vi "PathPlanner_PathFinder_WorkerThread.vi"() -> ()   [LabVIEW 2019]
uses:
  PathPlannerLib24/VI/PathPlanner_GridPosition_New.vi
  PathPlannerLib24/VI/PathPlanner_GridPosition_HashCode.vi
  PathPlannerLib24/VI/PathPlanner_PathFinder_Constants.vi
  PathPlannerLib24/VI/PathPlanner_PathFinder_Key.vi
  PathPlannerLib24/VI/PathPlanner_PathFinder_ClearOpen.vi
  PathPlannerLib24/VI/PathPlanner_PathFinder_ClearIncons.vi
  PathPlannerLib24/VI/PathPlanner_PathFinder_ClearClosed.vi
  PathPlannerLib24/VI/PathPlanner_PathFinder_ClearRHS.vi
  PathPlannerLib24/VI/PathPlanner_PathFinder_ClearG.vi
  PathPlannerLib24/VI/PathPlanner_PathFinder_ComputeOrImprovePath.vi
  PathPlannerLib24/VI/PathPlanner_PathFinder_SetNewPathAvail.vi
  PathPlannerLib24/VI/PathPlanner_PathFinder_ExtractPath.vi
  PathPlannerLib24/VI/PathPlanner_GridPosition_FromHash.vi
  PathPlannerLib24/VI/PathPlanner_GridPosition_Get.vi
  PathPlannerLib24/VI/PathPlanner_PathFinder_Heuristic.vi
  PathPlannerLib24/VI/PathPlanner_PathFinder_TopKey.vi
  PathPlannerLib24/VI/PathPlanner_PathFinder_ComparePair.vi
  PathPlannerLib24/VI/PathPlanner_PathFinder_UpdateState.vi
  PathPlannerLib24/VI/PathPlanner_PathFinder_GetOpenNeighbors.vi
  PathPlannerLib24/VI/PathPlanner_GridPosition_Equals.vi
  PathPlannerLib24/VI/PathPlanner_PathFinder_GridPosToTranslation2d.vi
  <vilib>/Rock Robotics/WPI/ThirdParty/JAS_Junk/TrajLib/Translation2d_GetDistance.vi
  <vilib>/Rock Robotics/WPI/ThirdParty/JAS_Junk/TrajLib/Translation2d_Create_DistAng.vi
  <vilib>/Rock Robotics/WPI/ThirdParty/JAS_Junk/TrajLib/Translation2d_Minus.vi
  <vilib>/Rock Robotics/WPI/ThirdParty/JAS_Junk/TrajLib/Translation2d_GetAngle.vi
  <vilib>/Rock Robotics/WPI/ThirdParty/JAS_Junk/TrajLib/Translation2d_Plus.vi
  PathPlannerLib24/VI/PathPlanner_PathFinder_ExtractPathSub1ALT.vi
  PathPlannerLib24/VI/PathPlanner_PathFinder_IsWalkable.vi
  PathPlannerLib24/VI/PathPlanner_PathFinder_Cost.vi
  <vilib>/Rock Robotics/WPI/ThirdParty/JAS_Junk/TrajLib/Translation2d_Create.vi
  <vilib>/Rock Robotics/WPI/ThirdParty/JAS_Junk/TrajLib/Util_CalcDist.vi
  <vilib>/Rock Robotics/WPI/ThirdParty/JAS_Junk/TrajLib/Rotation2d_GetAngleCosSin.vi
  <vilib>/Rock Robotics/WPI/ThirdParty/JAS_Junk/TrajLib/Translation2d_GetXY.vi
  <vilib>/Rock Robotics/WPI/ThirdParty/JAS_Junk/TrajLib/Rotation2d_CreateXY.vi
  PathPlannerLib24/VI/PathPlanner_PathFinder_IsCollision.vi
  PathPlannerLib24/VI/PathPlanner_GridPosition_Print.vi
  <vilib>/robotics/Navigation/shared/MapNode/AbstractDstarNode/NI_Robotics_AbstractDstarNode.lvclass
  C:/Program Files/National Instruments/LabVIEW 2019/vi.lib/robotics/Navigation/shared/MapNode/AbstractAstarNode/NI_Robotics_AbstractAstarNode.lvclass
  PathPlannerLib24/VI/PathPlanner_PathFinder_Globals.vi
  <vilib>/robotics/Navigation/shared/WorldMap/OccupancyGridWorldMap/Get Cells in Path.vi
  PathPlannerLib24/VI/PathPlanner_PathFinder_ApplyControlSmooth.vi
  PathPlannerLib24/VI/PathPlanner_PathFinder_ApplyAnchorSmooth.vi
  PathPlannerLib24/PathPlanner24.lvlib
panel:
  in  "Main Name":string
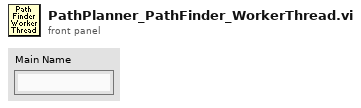
[diagram p1: front panel]
types:
  T1 = typedef "Semaphore RefNum" = refnum<k1>
  T2 = enum32{"Bad", "Idle", "Run top level", "Running"}
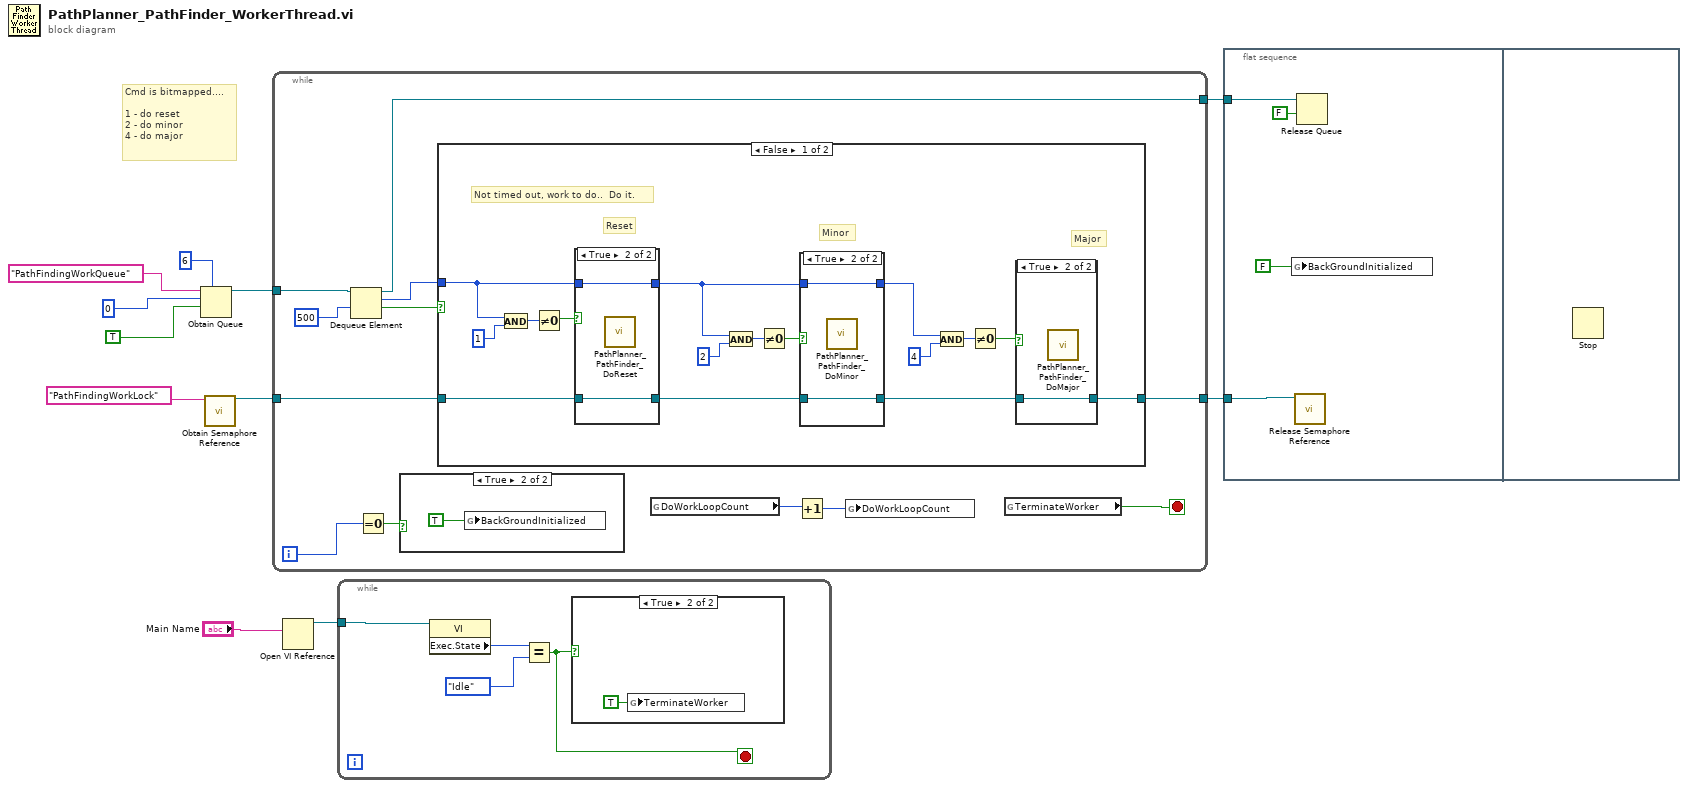
[diagram p0: block diagram]
diagram:
  # "Cmd is bitmapped....\n\n1 - do reset\n2 - do minor\n4 - do major"
  n1 = Obtain Queue(max queue size (-1, unlimited)=6, name (unnamed)="PathFindingWorkQueue", element data type=0, create if not found? (T)=TRUE) -> (queue out=w3:refnum<queue>)  [unwired: 1 in, 2 out]
  n2 = call <vilib>:"Obtain Semaphore Reference.vi"("name (unnamed)"="PathFindingWorkLock") -> ("semaphore"=w5:T1)  [unwired: 4 in, 2 out]
  n3 = while {
    tunnel: w3 -> [w22]
    tunnel: [w18] -> w7
    tunnel: w5 -> [w17]
    tunnel: [w16] -> w4
    i -> [w13]
    stop <- w23 stop-if-true
    n4 = Dequeue Element(queue=w22, timeout in ms (-1)=500) -> (queue out=w18:refnum<queue>, element=w19:i32, timed out?=w20:bool)  [unwired: 1 in, 1 out]
    n5 = Equal To 0?(x=w13) -> (x = 0?=w12:bool)
    n6 = case shown="True" w12 {
      frame False {
      }
      frame True {
        n7 = global write "PathPlanner_PathFinder_Globals.vi" "BackGroundInitialized"(TRUE ("TerminateWorker")) -> ()
      }
    }
    n8 = case shown="False" w20 {
      tunnel: w19 -> [w35 _]
      tunnel: w17 -> [w28 w51]
      tunnel: [w25 w51] -> w16
      frame False {
        # "Major"
        # "Minor"
        # "Reset"
        # "Not timed out, work to do..  Do it."
        n9 = And(x=w35, y=1) -> (x .and. y?=w38:i32)
        n10 = Not Equal To 0?(x=w38) -> (x != 0?=w39:bool)
        n11 = case shown="True" w39 {
          tunnel: w35 -> [w48 w50]
          tunnel: [w48 w50] -> w31
          tunnel: w28 -> [w47 w49]
          tunnel: [w47 w49] -> w27
          frame False {
          }
          frame True {
            n12 = call "PathPlanner_PathFinder_DoReset.vi"() -> ()  [unwired: 12 in]
          }
        }
        n13 = And(x=w31, y=2) -> (x .and. y?=w36:i32)
        n14 = Not Equal To 0?(x=w36) -> (x != 0?=w32:bool)
        n15 = case shown="True" w32 {
          tunnel: w31 -> [w44 w46]
          tunnel: [w44 w46] -> w29
          tunnel: w27 -> [w43 w45]
          tunnel: [w43 w45] -> w26
          frame False {
          }
          frame True {
            n16 = call "PathPlanner_PathFinder_DoMinor.vi"() -> ()  [unwired: 12 in]
          }
        }
        n17 = And(x=w29, y=4) -> (x .and. y?=w33:i32)
        n18 = Not Equal To 0?(x=w33) -> (x != 0?=w30:bool)
        n19 = case shown="True" w30 {
          tunnel: w26 -> [w41 w42]
          tunnel: [w41 w42] -> w25
          frame False {
          }
          frame True {
            n20 = call "PathPlanner_PathFinder_DoMajor.vi"() -> ()  [unwired: 12 in]
          }
        }
      }
      frame True {
        # "#TODO  Add I'm alive counter"
        # "Timed out, no work to do...."
      }
    }
    n21 = global read "PathPlanner_PathFinder_Globals.vi" "DoWorkLoopCount"() -> (w15:i64)
    n22 = Increment(x=w15) -> (x+1=w14:i64)
    n23 = global write "PathPlanner_PathFinder_Globals.vi" "DoWorkLoopCount"(w14) -> ()
    n24 = global read "PathPlanner_PathFinder_Globals.vi" "TerminateWorker"() -> (w23:bool)
  }
  n25 = Open VI Reference(vi path="Main Name") -> (vi reference=w1:refnum<vi>)  [unwired: 5 in, 1 out]
  n26 = while {
    tunnel: w1 -> [w52]
    stop <- w53 stop-if-true
    n27 = property class="VI"(reference=w52) -> ("Exec.State"=w55:T2)  [unwired: 1 in, 2 out]
    n28 = Equal?(x=w55, y=T2."Idle") -> (x = y?=w53:bool)
    n29 = case shown="True" w53 {
      frame False {
      }
      frame True {
        n30 = global write "PathPlanner_PathFinder_Globals.vi" "TerminateWorker"(TRUE ("TerminateWorker")) -> ()
      }
    }
  }
  n31 = flat-sequence {
    tunnel: w7 -> [w60]
    tunnel: w4 -> [w58]
    frame #0 {
      n32 = global write "PathPlanner_PathFinder_Globals.vi" "BackGroundInitialized"(FALSE ("TerminateWorker")) -> ()
      n33 = call <vilib>:"Release Semaphore Reference.vi"("semaphore"=w58) -> ()  [unwired: 9 in, 2 out]
      n34 = Release Queue(queue=w60, force destroy? (F)=FALSE) -> ()  [unwired: 1 in, 3 out]
    }
    frame #1 {
      n35 = Stop() -> ()  [unwired: 1 in]
    }
  }
